vi "Find Node By ID.vi"(8 "error in (no error)":errorcluster, 10 "Node Info":T1, 11 "ParseSVG in":refnum<class "ParseSVG.lvclass">) -> (0 "error out":errorcluster, 2 "Corrected XML":string, 3 "ParseSVG out":refnum<class "ParseSVG.lvclass">)   [LabVIEW 2019, in "ParseSVG.lvclass"]
uses:
  ParseSVG.lvclass
  ParseSVG.lvclass/ParseSVG.ctl
  <vilib>/xml/Close Reference(Node).vi
  <vilib>/xml/NI_XML.lvlib
  <resource>/objmgr/DOMUserDefRef.rc
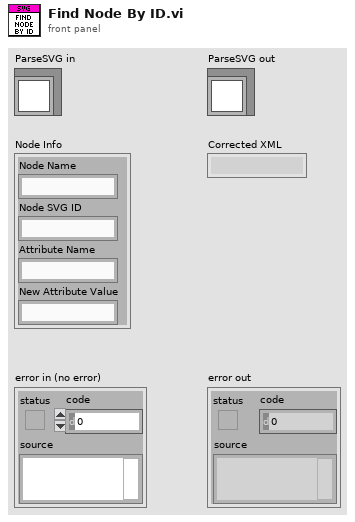
[diagram p1: front panel]
types:
  T1 = cluster{"Node Name":string, "Node SVG ID":string, "Attribute Name":string, "New Attribute Value":string}
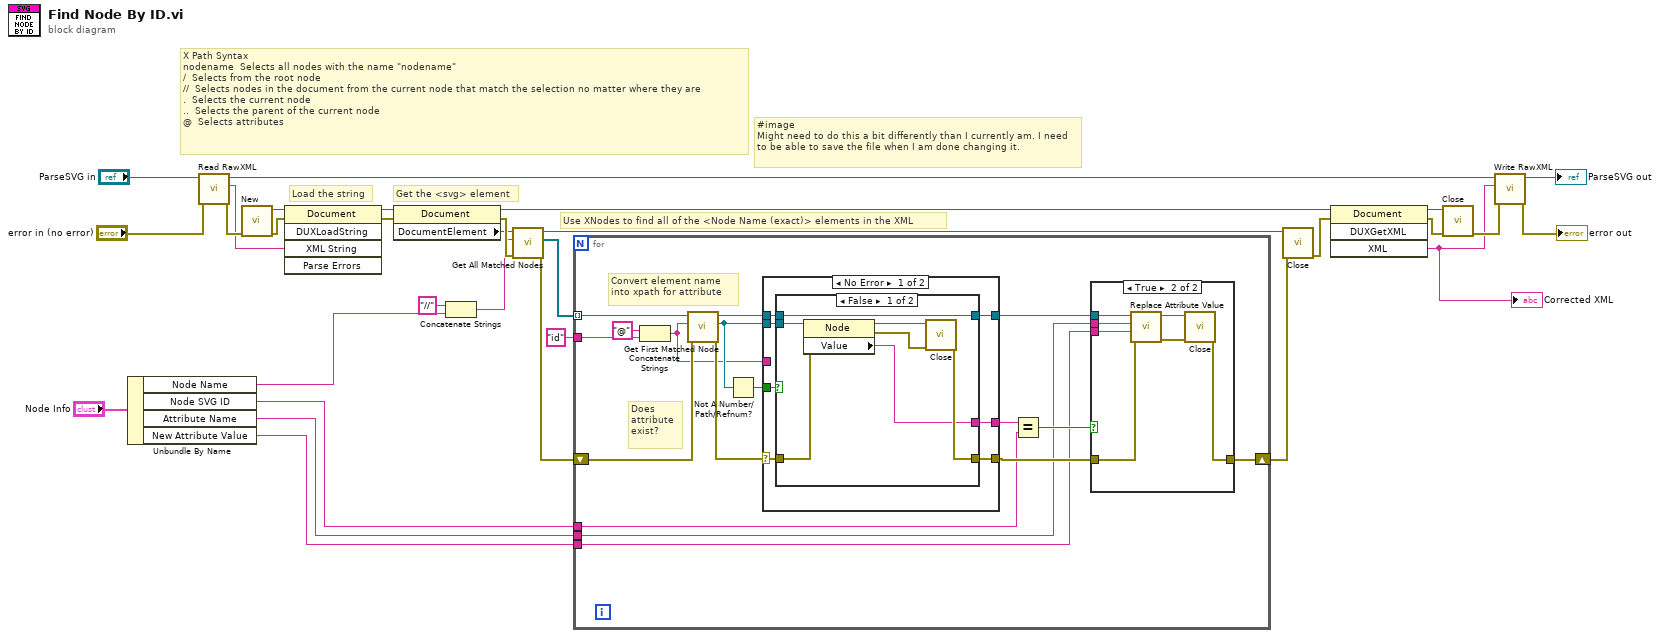
[diagram p0: block diagram]
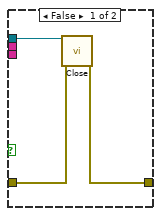
[diagram p2: hidden frame]
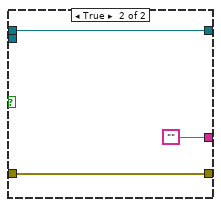
[diagram p3: hidden frame]
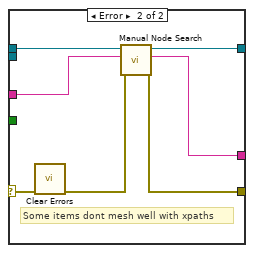
[diagram p4: hidden frame]
diagram:
  # "#image\nMight need to do this a bit differently than I currently am. I need to be able to save the file when I am done changing it."
  # "X Path Syntax\nnodename \tSelects all nodes with the name \"nodename\"\n/ \tSelects from the root node\n// \tSelects nodes in the document from the current node that match the selection no matter where they are\n. \tSelects the current node\n.. \tSelects the parent of the current node\n@ \tSelects attributes"
  # "Use XNodes to find all of the <Node Name (exact)> elements in the XML"
  # "Get the <svg> element"
  # "Load the string"
  n1 = Unbundle By Name("Node Info") -> ("Node Name"=w13:string, "Node SVG ID"=w12:string, "Attribute Name"=w11:string, "New Attribute Value"=w10:string)
  n2 = call "Read RawXML.vi"("error in (no error)"="error in (no error)", "ParseXML in"="ParseSVG in") -> ("error out"=w30:errorcluster, "RawXML"=w19:string, "ParseXML out"=w5:refnum<class "ParseSVG.lvclass">)  [unwired: 7 in]
  n3 = call <vilib>:"New.vi"("error in (no error)"=w30) -> ("error out"=w29:errorcluster, "DOM document out"=w26:refnum<k20>)  [unwired: 7 in]
  n4 = invoke class="Document" method="DUXLoadString"(reference=w26, error in=w29, "XML String"=w19) -> (reference out=w25:refnum<k20>, error out=w28:errorcluster)  [unwired: 2 in, 3 out]
  n5 = property class="Document"(reference=w25, error in=w28) -> (reference out=w9:refnum<k20>, error out=w27:errorcluster, "DocumentElement"=w24:refnum<k20>)
  n6 = Concatenate Strings("//" ("string"), w13) -> (w21:string)
  n7 = call <vilib>:"Get All Matched Nodes.vi"("error in (no error)"=w27, "XPath expression"=w21, "node in"=w24) -> ("error out"=w15:errorcluster, "node result array"=w22:refnum<k20>[], "node out"=w23:refnum<k20>)  [unwired: 6 in]
  n8 = for {
    tunnel: w22 -> [w46] mode=indexing
    shift-right: [w44] -> w31
    shift-left: w15 -> [w47]
    tunnel: "id" -> [w43]
    tunnel: w12 -> [w35]
    tunnel: w11 -> [w33]
    tunnel: w10 -> [w32]
    # "Convert element name into xpath for attribute"
    # "Does attribute exist?"
    n9 = Concatenate Strings("@" ("string"), w43) -> (w37:string)
    n10 = call <vilib>:"Get First Matched Node.vi"("error in (no error)"=w47, "XPath expression"=w37, "node in"=w46) -> ("error out"=w42:errorcluster, "node result"=w41:refnum<k20>, "node out"=w39:refnum<k20>)  [unwired: 6 in]
    n11 = Not A Number/Path/Refnum?(number/path/refnum=w41) -> (NaN/Path/Refnum?=w40:bool)
    n12 = case shown="No Error" w42 {
      selector: w42 -> [w64 w81]
      tunnel: [w65 w82] -> w48
      tunnel: w41 -> [w63 _]
      tunnel: w40 -> [w62 _]
      tunnel: w39 -> [w61 w78]
      tunnel: [w60 w79] -> w45
      tunnel: [w59 w76] -> w36
      tunnel: w37 -> [_ w77]
      frame No Error {
        n13 = case shown="False" w62 {
          tunnel: w64 -> [w72 w75]
          tunnel: [w71 w75] -> w65
          tunnel: w63 -> [w69 _]
          tunnel: w61 -> [w68 w74]
          tunnel: [w68 w74] -> w60
          tunnel: [w67 ""] -> w59
          frame False {
            n14 = property class="Node"(reference=w69, error in=w72) -> (reference out=w70:refnum<k20>, error out=w66:errorcluster, "Value"=w67:string)
            n15 = call-poly <vilib>:"Close.vi"("error in (no error)"=w66, "node"=w70) -> ("error out"=w71:errorcluster)  [unwired: 7 in]
          }
          frame True {
          }
        }
      }
      frame Error {
        # "Some items dont mesh well with xpaths"
        n16 = call <vilib>:"Clear Errors.vi"("error in (no error)"=w81) -> ("error out"=w80:errorcluster)  [unwired: 5 in, 1 out]
        n17 = call "Manual Node Search.vi"("error in (no error)"=w80, "XPath Syntax"=w77, "Node in"=w78) -> ("error out"=w82:errorcluster, "Value"=w76:string, "Node out"=w79:refnum<k20>)  [unwired: 6 in]
      }
    }
    n18 = Equal?(x=w36, y=w35) -> (x = y?=w34:bool)
    n19 = case shown="True" w34 {
      tunnel: w48 -> [w50 w53]
      tunnel: w45 -> [w51 w58]
      tunnel: [w49 w52] -> w44
      tunnel: w33 -> [_ w57]
      tunnel: w32 -> [_ w56]
      frame False {
        n20 = call-poly <vilib>:"Close.vi"("error in (no error)"=w50, "node"=w51) -> ("error out"=w49:errorcluster)  [unwired: 7 in]
      }
      frame True {
        n21 = call "Replace Attribute Value.vi"("error in (no error)"=w53, "New Value"=w56, "Attribute Name"=w57, "node in"=w58) -> ("error out"=w54:errorcluster, "Node Out"=w55:refnum<k20>)  [unwired: 6 in]
        n22 = call-poly <vilib>:"Close.vi"("error in (no error)"=w54, "node"=w55) -> ("error out"=w52:errorcluster)  [unwired: 7 in]
      }
    }
  }
  n23 = call-poly <vilib>:"Close.vi"("error in (no error)"=w31, "node"=w23) -> ("error out"=w7:errorcluster)  [unwired: 7 in]
  n24 = invoke class="Document" method="DUXGetXML"(reference=w9, error in=w7) -> (reference out=w8:refnum<k20>, error out=w6:errorcluster, "XML"=w1:string)  [unwired: 2 in, 1 out]
  "Corrected XML" <- w1
  n25 = call-poly <vilib>:"Close.vi"("error in (no error)"=w6, "node"=w8) -> ("error out"=w3:errorcluster)  [unwired: 7 in]
  n26 = call "Write RawXML.vi"("error in (no error)"=w3, "RawXML"=w1, "ParseSVG.lvclass"=w5) -> ("error out"=→"error out":errorcluster, "ParseSVG.lvclass 2"=→"ParseSVG out":refnum<class "ParseSVG.lvclass">)  [unwired: 7 in]
